vi "Get-timing-params.vi"(8 "error in (no error)":errorcluster, 11 "Acquis. params. ref. in":refnum<data-value>) -> (0 "error out":errorcluster, 1 "Period":i64, 2 "Source":string, 3 "Acquis. params. ref.":refnum<data-value>, 4 "Timeout":i32, 6 "Mode":T1=enum."Discard missed periods, ignore original phase")   [LabVIEW 2013, in "CameraVision.lvlib" / "CV-Acquisition.lvclass"]
uses:
  CV-Acquisition.lvclass
  <vilib>/Platform/TimedLoop/XDataNode/nitl_modes.ctl
  CV-Acquisition.lvclass/CV-Acquisition.ctl
  Read Timing source.vi
  Read Timing source period.vi
  Read Maximum frame rate.vi
  Read Minimum acquisition timeout.vi
  <vilib>/Platform/TimedLoop/XDataNode/XDNodeRunTimeDep.lvlib
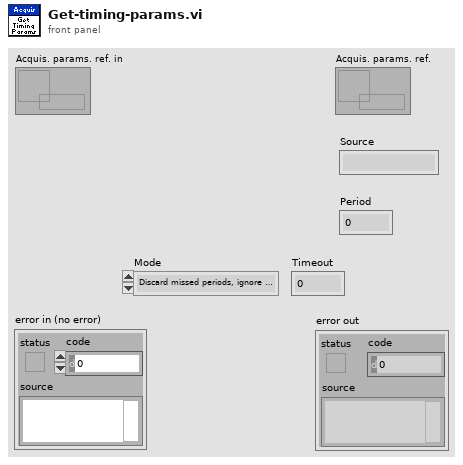
[diagram p1: front panel]
types:
  T1 = typedef "XDNodeRunTimeDep.lvlib/nitl_modes.ctl" = enum32{"No Change", "Process missed periods, maintain original phase", "Discard missed periods, maintain original phase", "Process missed periods, ignore original phase", "Discard missed periods, ignore original phase"}
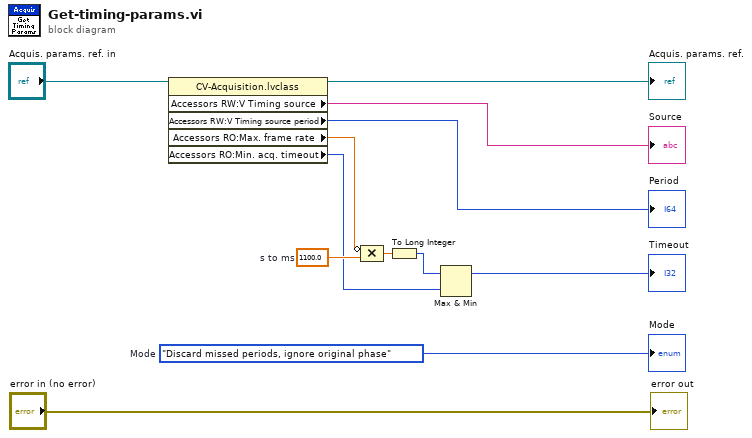
[diagram p0: block diagram]
diagram:
  w2 = nitl_modes."Discard missed periods, ignore original phase"  # Mode
  w8 = 1100.0  # s to ms
  n1 = property class="CV-Acquisition.lvclass"(reference="Acquis. params. ref. in") -> (reference out=→"Acquis. params. ref.":refnum<data-value>, "Accessors RW:V Timing source"=→"Source":string, "Accessors RW:V Timing source period"=→"Period":i64, "Accessors RO:Max. frame rate"=w9:dbl, "Accessors RO:Min. acq. timeout"=w1:i32)  [unwired: 1 in, 1 out]
  n2 = Compound Arithmetic op=MULTIPLY(invert w9, w8) -> (w7:dbl)
  n3 = To Long Integer(number=w7) -> (32bit integer=w6:i32)
  n4 = Max & Min(x=w6, y=w1) -> (max(x,y)=→"Timeout":i32)  [unwired: 1 out]
  "error out" <- "error in (no error)"
  "Mode" <- w2
